vi "Shoot Low Goal State Machine.vi"   [LabVIEW 2013]
uses:
  typedefs/fg_typedef.ctl
  typedefs/DevRef Type.ctl
  typedefs/State Machine/subStates.ctl
  typedefs/State Machine/singleUseSubstate.ctl
  <vilib>/Rock Robotics/WPI/Solenoid/WPI_SolenoidValue.ctl
  <vilib>/Rock Robotics/WPI/Solenoid/WPI_SolenoidGetEnum.vi
panel:
  # "A State Machine to Handle a Low Goal Shot"
types:
  T1 = typedef "DevRef Type.ctl" = enum16{"Shooter Solenoid", "Latch Solenoid", "Right Up Sensor", "Right Down Sensor", "Hold Sensor", "2 Ball Switch", "Arm Encoder"}
  T2 = typedef "fg_typedef.ctl" = enum16{"Get", "Set"}
  T3 = typedef "subStates.ctl" = enum16{"null", "wait", "driver control", "auto", "manual override", "hold position", "rotate", "pickup", "pass", "recover pass", "load", "goto shoot", "shoot high goal", "shoot low goal", "cancel arm", "cancel shooter", "end", "test"}
  T4 = typedef "WPI_SolenoidValue.ctl" = enum16{"Off", "On", "Forward", "Reverse"}
  T5 = typedef "singleUseSubstate.ctl" = enum16{"null", "wait", "shift high", "shift low", "extend shooter", "retract shooter", "latch", "unlatch", "end"}
  T6 = typedef "WPI_DigitalInputDevRef.ctl" = cluster{"DevStatus":errorcluster, "DIO Channel":T7, "Digital Module":T8}
  T7 = typedef "FPGA_DIOChannel.ctl" = enum8{"DIO 1", "DIO 2", "DIO 3", "DIO 4", "DIO 5", "DIO 6", "DIO 7", "DIO 8", "DIO 9", "DIO 10", "DIO 11", "DIO 12", "DIO 13", "DIO 14", "Invalid"}
  T8 = typedef "FPGA_TypedefDigitalModule.ctl" = enum16{"Digital Module 1", "Digital Module 2"}
  T9 = typedef "WPI_SolenoidDevRef.ctl" = cluster{"DevStatus":errorcluster, "Solenoid Module":T10, "Forward Solenoid Channel":T11, "Reverse Solenoid Channel":T11}
  T10 = typedef "FPGA_TypedefSolenoidModule.ctl" = enum16{"Solenoid Module 1", "Solenoid Module 2"}
  T11 = typedef "WPI_SolenoidChannel.ctl" = enum8{"Solenoid 1", "Solenoid 2", "Solenoid 3", "Solenoid 4", "Solenoid 5", "Solenoid 6", "Solenoid 7", "Solenoid 8", "Invalid"}
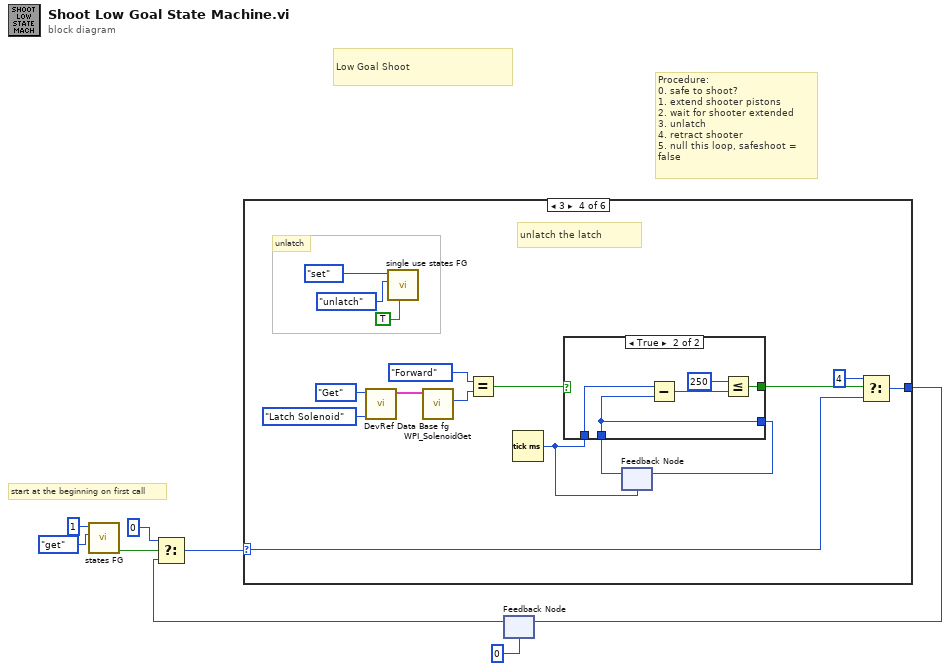
[diagram p0: block diagram]
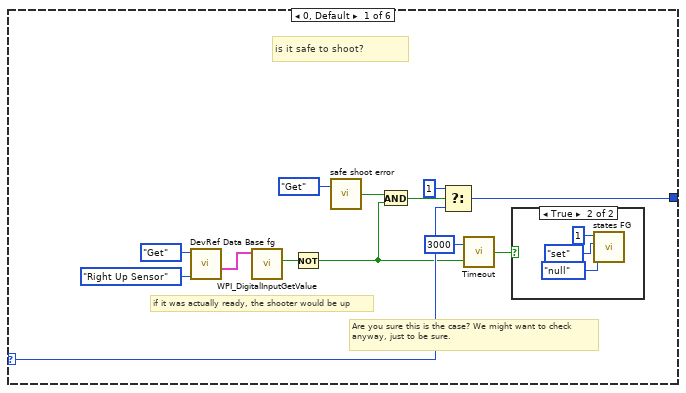
[diagram p2: hidden frame]
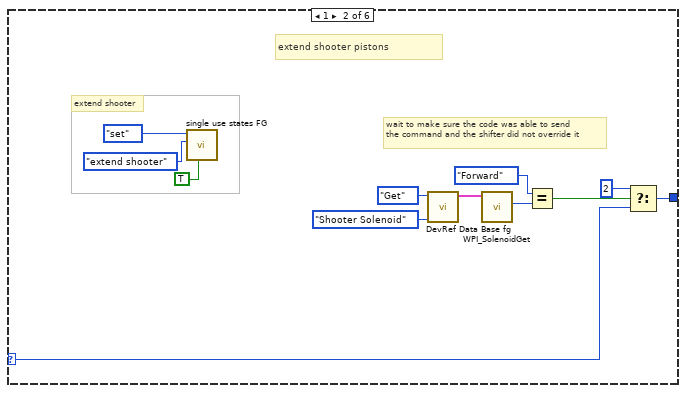
[diagram p4: hidden frame]
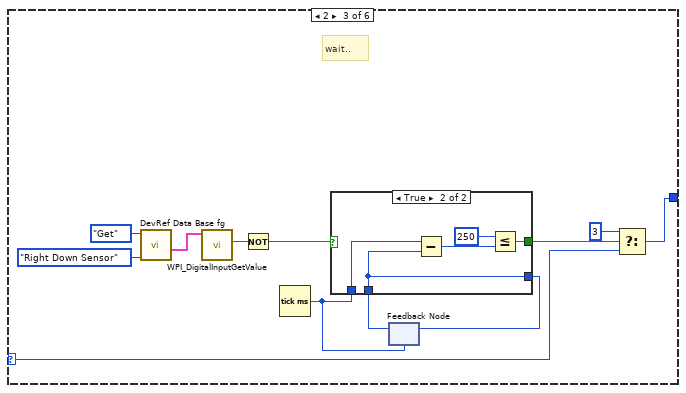
[diagram p5: hidden frame]
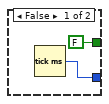
[diagram p6: hidden frame]
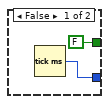
[diagram p7: hidden frame]
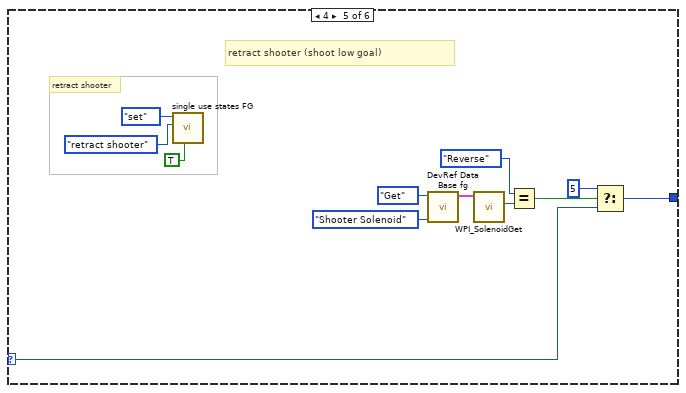
[diagram p8: hidden frame]
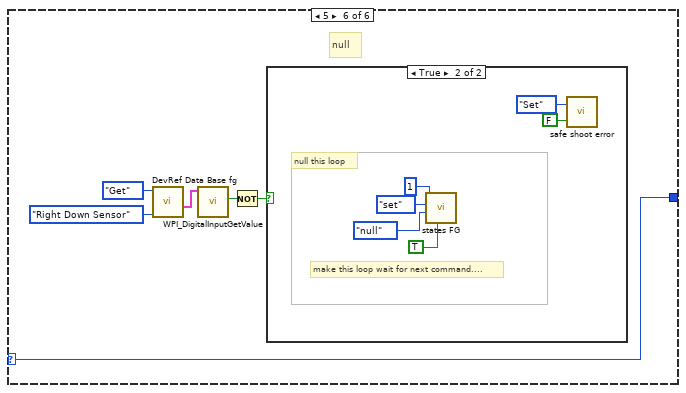
[diagram p9: hidden frame]
diagram:
  # "start at the beginning on first call"
  # "Low Goal Shoot"
  # "Procedure:\n0. safe to shoot? \n1. extend shooter pistons\n2. wait for shooter extended\n3. unlatch\n4. retract shooter\n5. null this loop, safeshoot = false"
  n1 = call "states FG.vi"("menu (get)"=enum16{"set", "get"}."get", "Loop ID"=1) -> ("first call?"=w1:bool)  [unwired: 6 in, 3 out]
  n2 = feedback #1(u8 0) -> (w4:u8)
  n3 = Select(t=u8 0, s=w1, f=w4) -> (s? t:f=w3:u8)
  n4 = case shown="3" w3 {
    selector: w3 -> [w14 w33 w47 w67 w82 w96]
    tunnel: [w19 w32 w46 w68 w83 w96] -> w7
    frame 0, Default {
      # "Are you sure this is the case? We might want to check\nanyway, just to be sure."
      # "if it was actually ready, the shooter would be up"
      # "is it safe to shoot?"
      n5 = call "DevRef Data Base fg.vi"("DevRef to Get"=DevRef_Type."Right Up Sensor", "Menu"=fg_typedef."Get") -> ("Selected Sensor"=w16:T6)  [unwired: 2 in, 5 out]
      n6 = call <vilib>:"WPI_DigitalInputGetValue.vi"("DigitalInputDevRef"=w16) -> ("Value"=w17:bool)  [unwired: 8 in, 2 out]
      n7 = Not(x=w17) -> (.not. x?=w13:bool)
      n8 = call "safe shoot error.vi"("Menu"=fg_typedef."Get") -> ("Can Shoot Safely?"=w20:bool)  [unwired: 1 in]
      n9 = And(x=w20, y=w13) -> (x .and. y?=w15:bool)
      n10 = Select(t=u8 1, s=w15, f=w14) -> (s? t:f=w19:u8)
      n11 = call "Timeout.vi"("Done with Task?"=w13, "Timeout (ms)"=u32 3000) -> ("Timed Out?"=w11:bool)  [unwired: 1 in]
      n12 = case shown="True" w11 {
        frame False {
        }
        frame True {
          n13 = call "states FG.vi"("subState in"=subStates."null", "menu (get)"=enum16{"set", "get"}."set", "Loop ID"=1) -> ()  [unwired: 5 in, 4 out]
        }
      }
    }
    frame 1 {
      # "wait to make sure the code was able to send\nthe command and the shifter did not override it"
      # "extend shooter"
      # "extend shooter pistons"
      n14 = call "single use states FG.vi"("exit in"=TRUE, "substate"=singleUseSubstate."extend shooter", "menu (get)"=enum16{"set", "get"}."set") -> ()  [unwired: 5 in, 4 out]
      n15 = call "DevRef Data Base fg.vi"("DevRef to Get"=DevRef_Type."Shooter Solenoid", "Menu"=fg_typedef."Get") -> ("Selected Solenoid"=w31:T9)  [unwired: 2 in, 5 out]
      n16 = call-poly <vilib>:"WPI_SolenoidGet.vi"("SolenoidDevRef"=w31) -> ("Value"=w30:T4)  [unwired: 8 in, 2 out]
      n17 = Equal?(x=WPI_SolenoidValue."Forward" ("Value"), y=w30) -> (x = y?=w28:bool)
      n18 = Select(t=u8 2, s=w28, f=w33) -> (s? t:f=w32:u8)
    }
    frame 2 {
      # "wait.."
      n19 = call "DevRef Data Base fg.vi"("DevRef to Get"=DevRef_Type."Right Down Sensor", "Menu"=fg_typedef."Get") -> ("Selected Sensor"=w45:T6)  [unwired: 2 in, 5 out]
      n20 = call <vilib>:"WPI_DigitalInputGetValue.vi"("DigitalInputDevRef"=w45) -> ("Value"=w48:bool)  [unwired: 8 in, 2 out]
      n21 = Not(x=w48) -> (.not. x?=w38:bool)
      n22 = Tick Count (ms)() -> (millisecond timer value=w39:u32)
      n23 = feedback #2(w39) -> (w40:u32)
      n24 = case shown="True" w38 {
        tunnel: w39 -> [_ w53]
        tunnel: [w50 w51] -> w41
        tunnel: w40 -> [_ w51]
        tunnel: [FALSE w52] -> w37
        frame False {
          n25 = Tick Count (ms)() -> (millisecond timer value=w50:u32)
        }
        frame True {
          n26 = Subtract(x=w53, y=w51) -> (x-y=w55:u32)
          n27 = Less Or Equal?(x=u32 250, y=w55) -> (x <= y?=w52:bool)
        }
      }
      n28 = feedback-in #2(w41) -> ()
      n29 = Select(t=u8 3, s=w37, f=w47) -> (s? t:f=w46:u8)
    }
    frame 3 {
      # "unlatch the latch"
      # "unlatch"
      n30 = call "DevRef Data Base fg.vi"("DevRef to Get"=DevRef_Type."Latch Solenoid", "Menu"=fg_typedef."Get") -> ("Selected Solenoid"=w66:T9)  [unwired: 2 in, 5 out]
      n31 = call "single use states FG.vi"("exit in"=TRUE, "substate"=singleUseSubstate."unlatch", "menu (get)"=enum16{"set", "get"}."set") -> ()  [unwired: 5 in, 4 out]
      n32 = call-poly <vilib>:"WPI_SolenoidGet.vi"("SolenoidDevRef"=w66) -> ("Value"=w65:T4)  [unwired: 8 in, 2 out]
      n33 = Equal?(x=WPI_SolenoidValue."Forward" ("Value"), y=w65) -> (x = y?=w57:bool)
      n34 = Tick Count (ms)() -> (millisecond timer value=w58:u32)
      n35 = feedback #3(w58) -> (w59:u32)
      n36 = case shown="True" w57 {
        tunnel: w58 -> [_ w76]
        tunnel: [w73 w74] -> w60
        tunnel: w59 -> [_ w74]
        tunnel: [FALSE w75] -> w56
        frame False {
          n37 = Tick Count (ms)() -> (millisecond timer value=w73:u32)
        }
        frame True {
          n38 = Subtract(x=w76, y=w74) -> (x-y=w78:u32)
          n39 = Less Or Equal?(x=u32 250, y=w78) -> (x <= y?=w75:bool)
        }
      }
      n40 = feedback-in #3(w60) -> ()
      n41 = Select(t=u8 4, s=w56, f=w67) -> (s? t:f=w68:u8)
    }
    frame 4 {
      # "retract shooter"
      # "retract shooter (shoot low goal)"
      n42 = call "single use states FG.vi"("exit in"=TRUE, "substate"=singleUseSubstate."retract shooter", "menu (get)"=enum16{"set", "get"}."set") -> ()  [unwired: 5 in, 4 out]
      n43 = call "DevRef Data Base fg.vi"("DevRef to Get"=DevRef_Type."Shooter Solenoid", "Menu"=fg_typedef."Get") -> ("Selected Solenoid"=w87:T9)  [unwired: 2 in, 5 out]
      n44 = call-poly <vilib>:"WPI_SolenoidGet.vi"("SolenoidDevRef"=w87) -> ("Value"=w86:T4)  [unwired: 8 in, 2 out]
      n45 = Equal?(x=WPI_SolenoidValue."Reverse" ("Value"), y=w86) -> (x = y?=w84:bool)
      n46 = Select(t=u8 5, s=w84, f=w82) -> (s? t:f=w83:u8)
    }
    frame 5 {
      # "null"
      n47 = call "DevRef Data Base fg.vi"("DevRef to Get"=DevRef_Type."Right Down Sensor", "Menu"=fg_typedef."Get") -> ("Selected Sensor"=w95:T6)  [unwired: 2 in, 5 out]
      n48 = call <vilib>:"WPI_DigitalInputGetValue.vi"("DigitalInputDevRef"=w95) -> ("Value"=w94:bool)  [unwired: 8 in, 2 out]
      n49 = Not(x=w94) -> (.not. x?=w93:bool)
      n50 = case shown="True" w93 {
        frame False {
        }
        frame True {
          # "null this loop"
          # "make this loop wait for next command...."
          n51 = call "states FG.vi"("exit in"=TRUE, "subState in"=subStates."null", "menu (get)"=enum16{"set", "get"}."set", "Loop ID"=1) -> ()  [unwired: 4 in, 4 out]
          n52 = call "safe shoot error.vi"("Can Shoot Safely?"=FALSE, "Menu"=fg_typedef."Set") -> ()  [unwired: 1 out]
        }
      }
    }
  }
  n53 = feedback-in #1(w7) -> ()
